vi "SwerveModuleOdometry.vi"(4 "Robot Heading(deg)":dbl, 5 "Module Fault":bool, 6 "Wheel Distance (in)":dbl, 7 "Wheel Azimuth (deg)":dbl, 9 "Velocity (ft/s)":dbl) -> (0 "Delta Y (in)":dbl, 1 "Delta X (in)":dbl, 2 "Velocity Y (ft/s)":dbl, 3 "Velocity X (ft/s)":dbl)   [LabVIEW 2019]
doc: "This VI calculates the field-centric delta odometry and velocity vectors for a single swerve module."
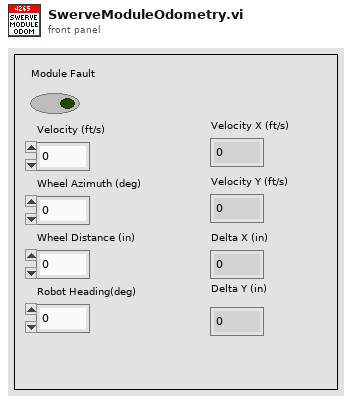
[diagram p1: front panel]
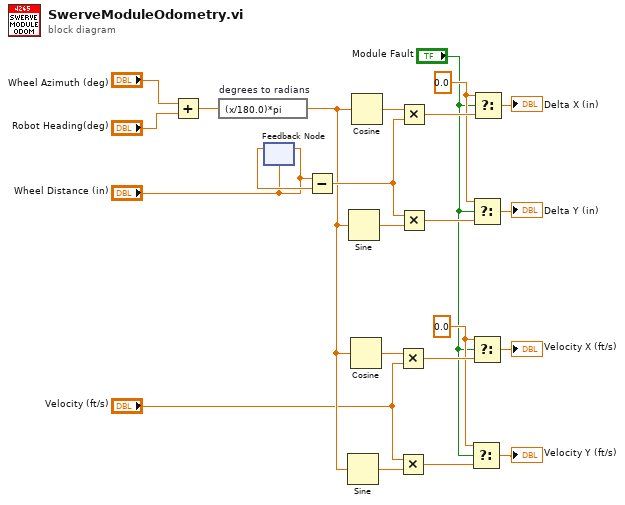
[diagram p0: block diagram]
diagram:
  w6 = 0.0 ("t")
  w13 = 0.0 ("t")
  n1 = Add(x="Wheel Azimuth (deg)", y="Robot Heading(deg)") -> (x+y=w18:dbl)
  n2 = expression code="(x/180.0)*pi" "degrees to radians"(w18) -> (w2:dbl)
  n3 = feedback #1("Wheel Distance (in)") -> (w12:dbl)
  n4 = feedback-in #1("Wheel Distance (in)") -> ()
  n5 = Subtract(x="Wheel Distance (in)", y=w12) -> (x-y=w20:dbl)
  n6 = Sine(x=w2) -> (sin(x)=w10:dbl)
  n7 = Sine(x=w2) -> (sin(x)=w21:dbl)
  n8 = Cosine(x=w2) -> (cos(x)=w9:dbl)
  n9 = Cosine(x=w2) -> (cos(x)=w19:dbl)
  n10 = Multiply(x=w9, y="Velocity (ft/s)") -> (x*y=w8:dbl)
  n11 = Multiply(x="Velocity (ft/s)", y=w10) -> (x*y=w7:dbl)
  n12 = Multiply(x=w19, y=w20) -> (x*y=w15:dbl)
  n13 = Multiply(x=w20, y=w21) -> (x*y=w14:dbl)
  n14 = Select(t=w6, s="Module Fault", f=w7) -> (s? t:f=→"Velocity Y (ft/s)":dbl)
  n15 = Select(t=w13, s="Module Fault", f=w14) -> (s? t:f=→"Delta Y (in)":dbl)
  n16 = Select(t=w6, s="Module Fault", f=w8) -> (s? t:f=→"Velocity X (ft/s)":dbl)
  n17 = Select(t=w13, s="Module Fault", f=w15) -> (s? t:f=→"Delta X (in)":dbl)
